vi "HIOKI PW3390 Conf CH B DC.vi"(0 "VISA Resource":refnum<visa-resource-name>, 1 "Range (1: 5V)":enum16{"1", "5", "10"}(ring)=enum."5", 3 "Scaling (1.00)":dbl=1.0 min=0.01 max=9999.99 format="%.2f", 4 "Motorpoles (4)":i32=4 min=2 max=98 step=2, 5 "error in (no error)":errorcluster, 6 "Set/Query (F: Set)":bool, 7 "Unit (2: rpm)":enum16{"V", "Hz", "rpm"}(ring)=enum."rpm", 9 "OPC query (T: ON)":bool=TRUE, 11 "Error Out (F: Off)":bool) -> (12 "CH B input out":enum16{"PULSE", "DC"}(ring)=enum."DC", 13 "Unit out":enum16{"V", "Hz", "rpm"}(ring)=enum."rpm", 14 "VISA Resource out":refnum<visa-resource-name>, 15 "Range out":enum16{"1", "5", "10"}(ring)=enum."5", 17 "Scaling out":dbl=1.0 format="%.2f", 18 "Motorpoles out":i32=4, 19 "error out":errorcluster)   [LabVIEW 2009]
doc: "Sets and reads the functions related to the Motor Analysis Option's Channel B voltage.\n\nSet/Query\n Set: Send the setting commands for the device.\n Query: Query the setting of the device.\n\nRange\n Sets the voltage range of Channel B.\n\nScaling\n Sets the Scaling of Channel B.\n Input Range: 0. 01 - 9999.99\n\nMotorpoles\n Sets the Motor Poles. When an odd number is set, an even number smaller than the set value will be set.\n Input Range: even values of 2 - 98\n\nUnit\n Sets the unit of Channel B."
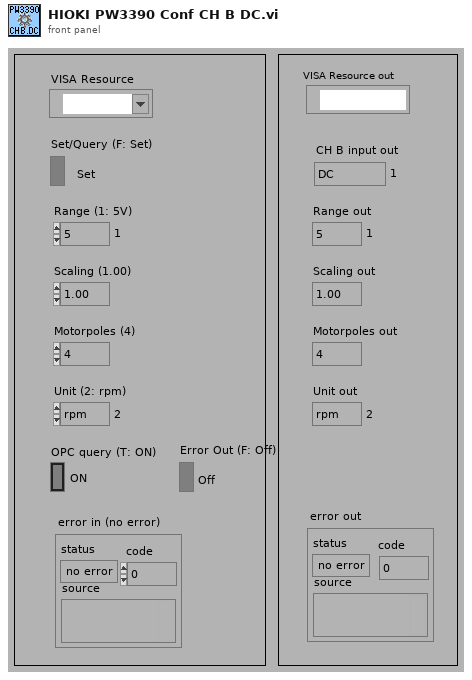
[diagram p1: front panel]
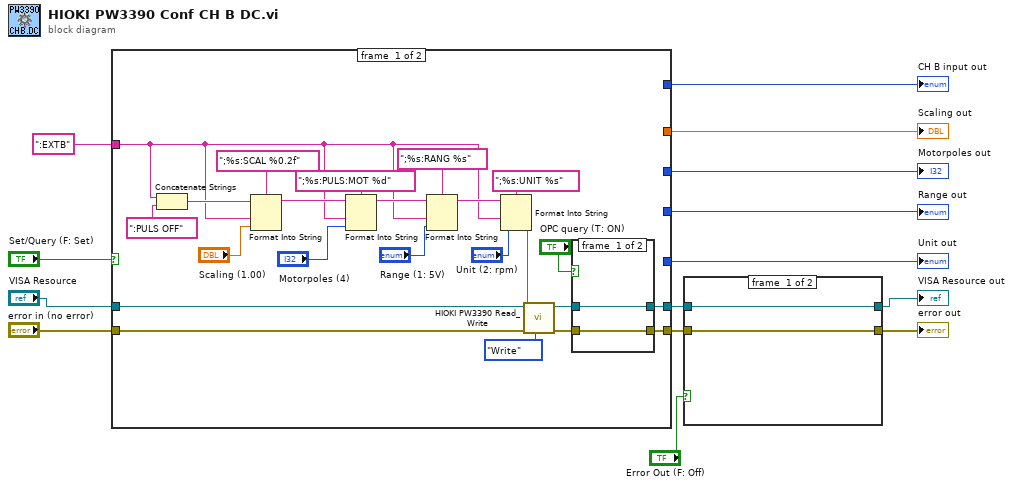
[diagram p0: block diagram]
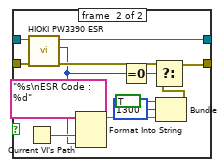
[diagram p2: hidden frame]
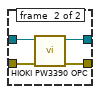
[diagram p3: hidden frame]
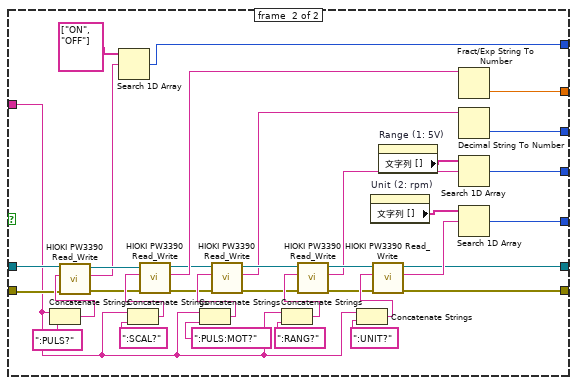
[diagram p4: hidden frame]
diagram:
  n1 = case shown="FALSE" "Set/Query (F: Set)" {
    tunnel: "error in (no error)" -> [w33 w51]
    tunnel: [w18 w67] -> w7
    tunnel: "VISA Resource" -> [w34 w52]
    tunnel: [w19 w68] -> w6
    tunnel: [_ w66] -> w12
    tunnel: ":EXTB" -> [w16 w48]
    tunnel: [_ w62] -> w10
    tunnel: [_ w76] -> w9
    tunnel: [_ w54] -> w4
    tunnel: [_ w44] -> w1
    frame #0 {
      n2 = Concatenate Strings(w16, ":PULS OFF") -> (w17:string)
      n3 = Format Into String(format string=";%s:SCAL %0.2f", initial string=w17, w16, "Scaling (1.00)") -> (resulting string=w24:string)  [unwired: 1 in, 1 out]
      n4 = Format Into String(format string=";%s:PULS:MOT %d", initial string=w24, w16, "Motorpoles (4)") -> (resulting string=w23:string)  [unwired: 1 in, 1 out]
      n5 = Format Into String(format string=";%s:RANG %s", initial string=w23, w16, "Range (1: 5V)") -> (resulting string=w29:string)  [unwired: 1 in, 1 out]
      n6 = Format Into String(format string=";%s:UNIT %s", initial string=w29, w16, "Unit (2: rpm)") -> (resulting string=w27:string)  [unwired: 1 in, 1 out]
      n7 = call <instrlib>:"HIOKI PW3390 Read_Write.vi"("Read/Write"=enum16{"Read", "Write"}."Write", "error in (no error)"=w33, "data in"=w27, "VISA Resource"=w34) -> ("error out"=w20:errorcluster, "VISA Resource out"=w21:refnum<visa-resource-name>)  [unwired: 5 in, 1 out]
      n8 = case shown="TRUE" "OPC query (T: ON)" {
        tunnel: [w39 w43] -> w19
        tunnel: [w38 w42] -> w18
        tunnel: w21 -> [w39 w41]
        tunnel: w20 -> [w38 w40]
        frame #0 {
        }
        frame #1 {
          n9 = call <instrlib>:"HIOKI PW3390 OPC.vi"("error in (no error)"=w40, "VISA Resource"=w41) -> ("error out"=w42:errorcluster, "VISA Resource out"=w43:refnum<visa-resource-name>)  [unwired: 7 in, 1 out]
        }
      }
    }
    frame #1 {
      n10 = Concatenate Strings(w48, ":PULS?" ("文字列")) -> (w53:string)
      n11 = call <instrlib>:"HIOKI PW3390 Read_Write.vi"("error in (no error)"=w51, "data in"=w53, "VISA Resource"=w52) -> ("error out"=w49:errorcluster, "data out"=w45:string, "VISA Resource out"=w50:refnum<visa-resource-name>)  [unwired: 6 in]
      n12 = Search 1D Array(1D array=string[] ["ON", "OFF"] ("文字列配列"), element=w45) -> (index of element=w44:i32)  [unwired: 1 in]
      n13 = Concatenate Strings(w48, ":SCAL?") -> (w73:string)
      n14 = call <instrlib>:"HIOKI PW3390 Read_Write.vi"("error in (no error)"=w49, "data in"=w73, "VISA Resource"=w50) -> ("error out"=w59:errorcluster, "data out"=w65:string, "VISA Resource out"=w56:refnum<visa-resource-name>)  [unwired: 6 in]
      n15 = Concatenate Strings(w48, ":PULS:MOT?") -> (w61:string)
      n16 = call <instrlib>:"HIOKI PW3390 Read_Write.vi"("error in (no error)"=w59, "data in"=w61, "VISA Resource"=w56) -> ("error out"=w58:errorcluster, "data out"=w55:string, "VISA Resource out"=w57:refnum<visa-resource-name>)  [unwired: 6 in]
      n17 = Concatenate Strings(w48, ":RANG?") -> (w75:string)
      n18 = call <instrlib>:"HIOKI PW3390 Read_Write.vi"("error in (no error)"=w58, "data in"=w75, "VISA Resource"=w57) -> ("error out"=w69:errorcluster, "data out"=w63:string, "VISA Resource out"=w70:refnum<visa-resource-name>)  [unwired: 6 in]
      n19 = Concatenate Strings(w48, ":UNIT?") -> (w74:string)
      n20 = property on="Unit (2: rpm)" class="Enum (strict)"() -> ("文字列 []"=w72:string[])  [unwired: 2 in, 2 out]
      n21 = call <instrlib>:"HIOKI PW3390 Read_Write.vi"("error in (no error)"=w69, "data in"=w74, "VISA Resource"=w70) -> ("error out"=w67:errorcluster, "data out"=w71:string, "VISA Resource out"=w68:refnum<visa-resource-name>)  [unwired: 6 in]
      n22 = property on="Range (1: 5V)" class="Enum (strict)"() -> ("文字列 []"=w64:string[])  [unwired: 2 in, 2 out]
      n23 = Fract/Exp String To Number(string=w65) -> (number=w66:dbl)  [unwired: 3 in, 1 out]
      n24 = Decimal String To Number(string=w55) -> (number=w54:i32)  [unwired: 2 in, 1 out]
      n25 = Search 1D Array(1D array=w64, element=w63) -> (index of element=w62:i32)  [unwired: 1 in]
      n26 = Search 1D Array(1D array=w72, element=w71) -> (index of element=w76:i32)  [unwired: 1 in]
    }
  }
  "Scaling out" <- w12
  "Unit out" <- w9
  "Range out" <- w10
  "Motorpoles out" <- w4
  "CH B input out" <- w1
  n27 = case shown="TRUE" "Error Out (F: Off)" {
    tunnel: w6 -> [w81 w94]
    tunnel: w7 -> [w80 w93]
    tunnel: [w80 w83] -> w5
    tunnel: [w81 w92] -> w2
    frame #0 {
    }
    frame #1 {
      n28 = Current VI's Path() -> (path=w90:path)
      n29 = call <instrlib>:"HIOKI PW3390 ESR.vi"("error in (no error)"=w93, "VISA Resource"=w94) -> ("error out"=w84:errorcluster, "Output Value"=w82:u8, "VISA Resource out"=w92:refnum<visa-resource-name>)  [unwired: 6 in, 1 out]
      n30 = Format Into String(format string="%s\nESR Code : %d", w90, w82) -> (resulting string=w86:string)  [unwired: 2 in, 1 out]
      n31 = Equal To 0?(x=w82) -> (x = 0?=w91:bool)
      n32 = Bundle("status"=TRUE, "code"=1300, w86) -> (w85:cluster{"status":bool, "code":i32, string})  [unwired: 1 in]
      n33 = Select(t=w84, s=w91, f=w85) -> (s? t:f=w83:errorcluster)
    }
  }
  "error out" <- w5
  "VISA Resource out" <- w2
